vi "FunctionGenerator_Calculate.vi"(9 "Input Value":dbl, 11 "FUNCTION_GENERATOR":T1) -> (3 "Output Value":dbl)   [LabVIEW 2019, in "Trajectory_Library.lvlib"]
doc: "Calculate the output Y value for the provided X. This is done by interpolating through an array of X and Y pairs. The pairs must be ordered in increasing X value.\n\nIf there's no matching key, the value returned will be a linear interpolation between the keys before and after the provided one.\n\n\nInputs:\n - Function_Generator -- function generator data structure\n - Input Value -- The input value. \n\nOutputs:\n - Output Value -- Output value calcuated from the input value."
uses:
  Trajectory_Library.lvlib
  TypeDef/FUNCTION_GENERATOR.ctl
  <vilib>/gmath/NI_Gmath.lvlib
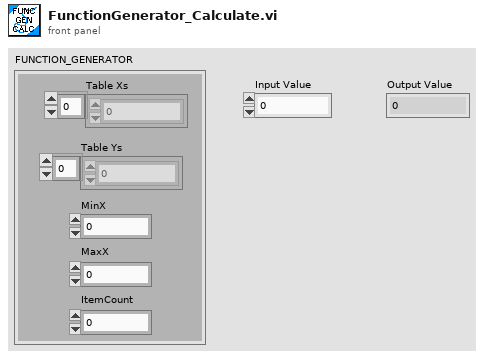
[diagram p1: front panel]
types:
  T1 = typedef "Trajectory_Library.lvlib/FUNCTION_GENERATOR.ctl" = cluster{"Table Xs":dbl[], "Table Ys":dbl[], "MinX":dbl, "MaxX":dbl, "ItemCount":i32}
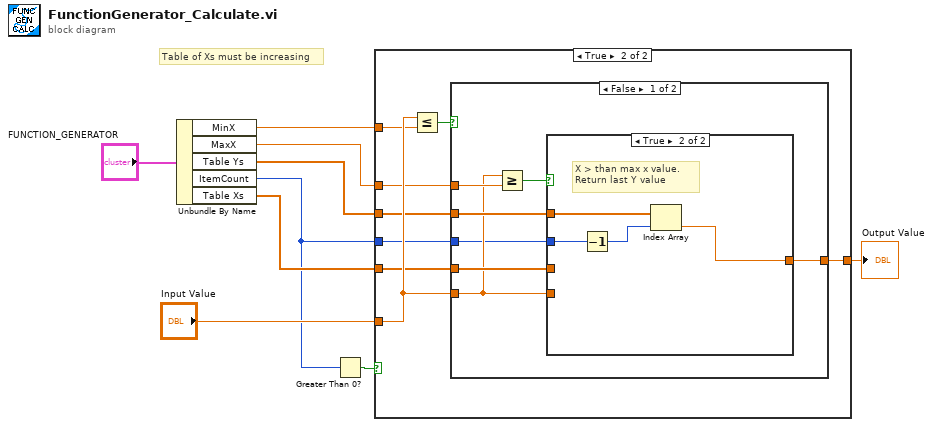
[diagram p0: block diagram]
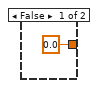
[diagram p2: hidden frame]
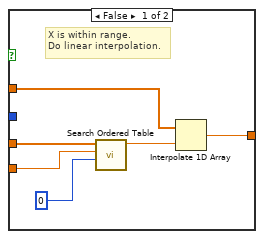
[diagram p3: hidden frame]
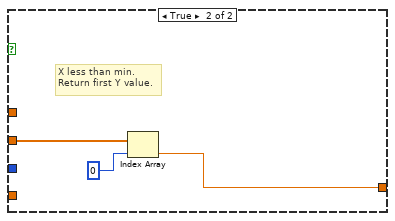
[diagram p4: hidden frame]
diagram:
  # "Table of Xs must be increasing"
  n1 = Unbundle By Name("FUNCTION_GENERATOR") -> ("MinX"=w6:dbl, "MaxX"=w5:dbl, "Table Ys"=w3:dbl[], "ItemCount"=w1:i32, "Table Xs"=w4:dbl[])
  n2 = Greater Than 0?(x=w1) -> (x > 0?=w2:bool)
  n3 = case shown="True" w2 {
    tunnel: "Input Value" -> [_ w17]
    tunnel: [0.0 ("Table Y") w16] -> w8
    tunnel: w6 -> [_ w15]
    tunnel: w5 -> [_ w14]
    tunnel: w1 -> [_ w13]
    tunnel: w4 -> [_ w12]
    tunnel: w3 -> [_ w11]
    frame False {
    }
    frame True {
      n4 = Less Or Equal?(x=w17, y=w15) -> (x <= y?=w18:bool)
      n5 = case shown="False" w18 {
        tunnel: w11 -> [w23 w38]
        tunnel: [w22 w36] -> w16
        tunnel: w17 -> [w20 _]
        tunnel: w14 -> [w25 _]
        tunnel: w12 -> [w21 _]
        tunnel: w13 -> [w19 _]
        frame False {
          n6 = Greater Or Equal?(x=w20, y=w25) -> (x >= y?=w24:bool)
          n7 = case shown="True" w24 {
            tunnel: w23 -> [w28 w35]
            tunnel: [w26 w34] -> w22
            tunnel: w21 -> [w30 _]
            tunnel: w20 -> [w29 _]
            tunnel: w19 -> [_ w33]
            frame False {
              # "X is within range.  \nDo linear interpolation."
              n8 = call <vilib>:"Search Ordered Table.vi"("starting index"=0, "x value"=w29, "ordered x array"=w30) -> ("fractional index"=w27:dbl)  [unwired: 8 in]
              n9 = Interpolate 1D Array(1:w27, 2:w28) -> (0:w26:dbl)
            }
            frame True {
              # "X > than max x value.   \nReturn last Y value"
              n10 = Decrement(x=w33) -> (x-1=w32:i32)
              n11 = Index Array(array=w35, index=w32) -> (element=w34:dbl)
            }
          }
        }
        frame True {
          # "X less than min.   \nReturn first Y value."
          n12 = Index Array(array=w38, index=0) -> (element=w36:dbl)
        }
      }
    }
  }
  "Output Value" <- w8
